vi "Agilent SNA Get Stimulus.vi"(7 "Agilent SNA & SWP":T2, 8 "error in (no error)":errorcluster, 9 "Channel":i8=1 min=1 max=99 step=1, 11 "VISA Resource Names":T1) -> (0 "error out":errorcluster, 2 "SP Stimulus":T3={"Use Instrument Settings"=FALSE, "Blank Frequencies"=FALSE, "Sweep Type"=enum."Linear", "Sweep"={"Fstart"=500.0, "Fstop"=1500.0, "Units"=enum."MHz", "Points"=201}, "Power (dBm)"=999.0, "IFBW (Hz)"=-1.0, "Sweep Time (s)"=-1.0, "Calibration"={"State"=FALSE, "String"=""}} {"Sweep Time (s)" format="%.3g"}, 3 "dup VISA Resource Names":T1)   [LabVIEW 2011]
uses:
  tests/S Parameter/TypeDefs/SP Stimulus Parameters.ctl
  tests/S Parameter/TypeDefs/SP Frequency Units.ctl
  tests/S Parameter/TypeDefs/SP Calibration State.ctl
  TypeDefs/Agilent SNA VISA.ctl
  TypeDefs/Agilent SNA Instrument Info.ctl
  TypeDefs/Agilent SNA Message Mode.ctl
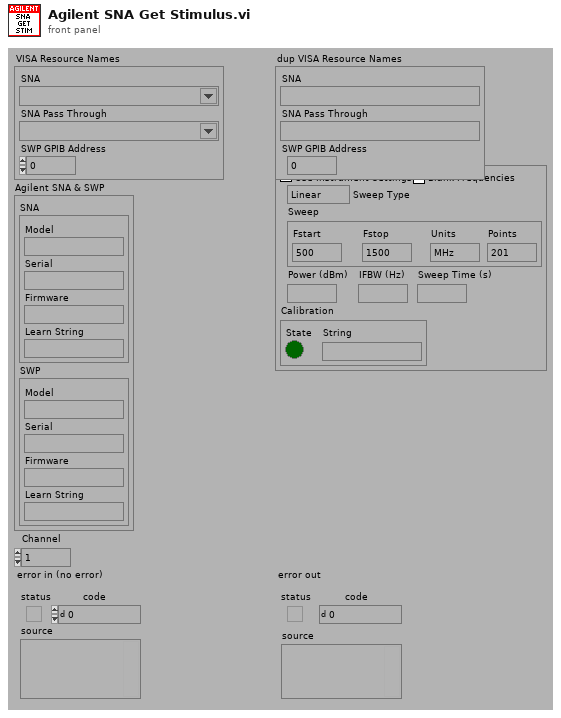
[diagram p1: front panel]
types:
  T1 = typedef "Agilent SNA VISA.ctl" = cluster{"SNA":refnum<visa-resource-name>, "SNA Pass Through":refnum<visa-resource-name>, "SWP GPIB Address":i32}
  T2 = typedef "Agilent SNA Instrument Info.ctl" = cluster{"SNA":cluster{"Model":string, "Serial":string, "Firmware":string, "Learn String":string}, "SWP":cluster{"Model":string, "Serial":string, "Firmware":string, "Learn String":string}}
  T3 = typedef "SP Stimulus Parameters.ctl" = cluster{"Use Instrument Settings":bool, "Blank Frequencies":bool, "Sweep Type":enum32{"Linear", "Logarithmic", "List", "Power", "CW"}, "Sweep":cluster{"Fstart":dbl, "Fstop":dbl, "Units":T4, "Points":i32}, "Power (dBm)":dbl, "IFBW (Hz)":dbl, "Sweep Time (s)":dbl, "Calibration":T5}
  T4 = typedef "SP Frequency Units.ctl" = enum16{"Hz", "kHz", "MHz", "GHz", "Points"}
  T5 = typedef "SP Calibration State.ctl" = cluster{"State":bool, "String":string}
  T6 = typedef "Agilent SNA Message Mode.ctl" = enum16{"On", "Off"}
  T7 = typedef "Agilent SNA Sweep Type.ctl" = enum32{"Linear Sweep", "CW Time Sweep", "Frequency List"}
  T8 = enum32{"Linear", "Logarithmic", "List", "Power", "CW"}
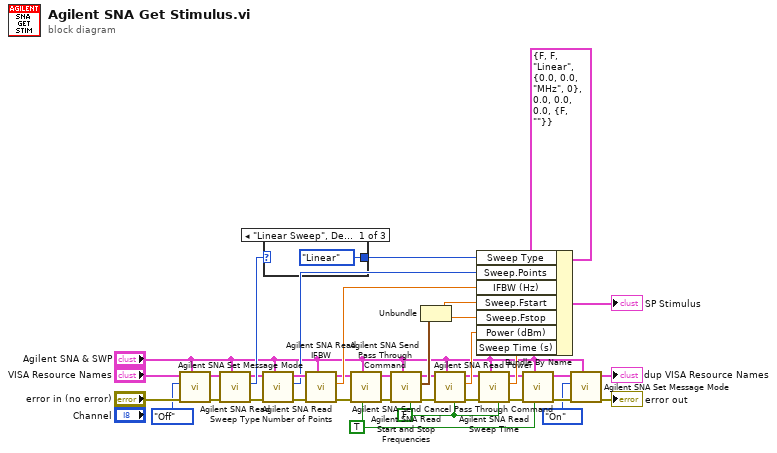
[diagram p0: block diagram]
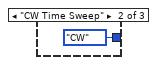
[diagram p2: hidden frame]
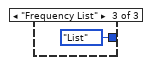
[diagram p3: hidden frame]
diagram:
  w12 = FALSE ("Passthrough (T)")
  w23 = TRUE ("SCPI? (F)")
  n1 = call "Agilent SNA Set Message Mode.vi"("Agilent SNA & SWP"="Agilent SNA & SWP", "error in (no error)"="error in (no error)", "Message Mode"=Agilent_SNA_Message_Mode."Off", "VISA Resource Names"="VISA Resource Names") -> ("error out"=w6:errorcluster, "dup VISA Resource Names"=w7:T1)  [unwired: 6 out]
  n2 = call "Agilent SNA Read Sweep Type.vi"("Agilent SNA & SWP"="Agilent SNA & SWP", "error in (no error)"=w6, "VISA Resource Names"=w7) -> ("error out"=w29:errorcluster, "Sweep Type"=w35:T7, "dup VISA Resource Names"=w32:T1)  [unwired: 1 in, 5 out]
  n3 = call "Agilent SNA Read Number of Points.vi"("Agilent SNA & SWP"="Agilent SNA & SWP", "error in (no error)"=w29, "VISA Resource Names"=w32) -> ("error out"=w30:errorcluster, "Number Points"=w28:i32, "dup VISA Resource Names"=w31:T1)  [unwired: 1 in, 5 out]
  n4 = case shown="\"Linear Sweep\", Default" w35 {
    tunnel: [T8."Linear" ("Sweep Type") T8."CW" ("Sweep Type") T8."List" ("Sweep Type")] -> w33
    frame "Linear Sweep", Default {
    }
    frame "CW Time Sweep" {
    }
    frame "Frequency List" {
    }
  }
  n5 = call "Agilent SNA Read IFBW.vi"("Agilent SNA & SWP"="Agilent SNA & SWP", "error in (no error)"=w30, "VISA Resource Names"=w31) -> ("error out"=w21:errorcluster, "IFBW, Hz"=w27:dbl, "dup VISA Resource Name"=w22:T1)  [unwired: 1 in, 5 out]
  n6 = call "Agilent SNA Send Pass Through Command.vi"("SCPI? (F)"=w23, "Agilent SNA & SWP"="Agilent SNA & SWP", "error in (no error)"=w21, "VISA Resource Names"=w22) -> ("error out"=w18:errorcluster, "dup VISA Resource Names"=w17:T1)  [unwired: 6 out]
  n7 = call "Agilent SNA Read Start and Stop Frequencies.vi"("Passthrough (T)"=w12, "Agilent SNA & SWP"="Agilent SNA & SWP", "error in (no error)"=w18, "VISA Resource Names"=w17) -> ("error out"=w13:errorcluster, "Start/Stop Freqs, MHz"=w34:cluster{"Fstart":dbl, "Fstop":dbl}, "dup VISA Resource Names"=w16:T1)  [unwired: 1 in, 4 out]
  n8 = Unbundle(w34) -> ("Fstart"=w25:dbl, "Fstop"=w26:dbl)
  n9 = call "Agilent SNA Read Power.vi"("Passthrough (T)"=w12, "Agilent SNA & SWP"="Agilent SNA & SWP", "error in (no error)"=w13, "VISA Resource Names"=w16) -> ("error out"=w14:errorcluster, "Source Power, dBm"=w24:dbl, "dup VISA Resource Names"=w15:T1)  [unwired: 1 in, 4 out]
  n10 = call "Agilent SNA Read Sweep Time.vi"("Passthrough (T)"=w12, "Agilent SNA & SWP"="Agilent SNA & SWP", "error in (no error)"=w14, "VISA Resource Names"=w15) -> ("error out"=w19:errorcluster, "Sweep Time, s"=w37:dbl, "dup VISA Resource Name"=w20:T1)  [unwired: 1 in, 4 out]
  n11 = Bundle By Name(cluster=T3 {"Use Instrument Settings"=FALSE, "Blank Frequencies"=FALSE, "Sweep Type"=enum."Linear", "Sweep"={"Fstart"=0.0, "Fstop"=0.0, "Units"=enum."MHz", "Points"=0}, "Power (dBm)"=0.0, "IFBW (Hz)"=0.0, "Sweep Time (s)"=0.0, "Calibration"={"State"=FALSE, "String"=""}} ("Stimulus"), "Sweep Type"=w33, "Sweep.Points"=w28, "IFBW (Hz)"=w27, "Sweep.Fstart"=w25, "Sweep.Fstop"=w26, "Power (dBm)"=w24, "Sweep Time (s)"=w37) -> (→"SP Stimulus":T3)
  n12 = call "Agilent SNA Send Cancel Pass Through Command.vi"("SCPI? (F)"=w23, "Agilent SNA & SWP"="Agilent SNA & SWP", "error in (no error)"=w19, "VISA Resource Names"=w20) -> ("error out"=w11:errorcluster, "dup VISA Resource Names"=w8:T1)  [unwired: 6 out]
  n13 = call "Agilent SNA Set Message Mode.vi"("Agilent SNA & SWP"="Agilent SNA & SWP", "error in (no error)"=w11, "Message Mode"=Agilent_SNA_Message_Mode."On", "VISA Resource Names"=w8) -> ("error out"=→"error out":errorcluster, "dup VISA Resource Names"=→"dup VISA Resource Names":T1)  [unwired: 6 out]
